vi "Bezier Trajectory.vi"(4 "Turn Rate":dbl=5.0 format="%#_13g", 5 "Max Robot Speed":dbl, 6 "Overrides":T3 {"Angle Override" step=5.0; "Velocity Override" step=5.0; "Angular Override" step=5.0}, 7 "Drive Type":T6, 8 "Conditions":T7, 9 "All Limits":cluster{"Limits":T4, "Angular Limits":T5} {"Limits"."StoopidFast (fps)" min=0.0; "Limits"."Jerk (fps^3)" min=0.0 step=1.0; "Limits"."Accel (fps^2)" min=0.0; "Limits"."Velocity (fps)" min=0.0; "Angular Limits"."Jerk (deg/s^3)" min=0.0 step=1.0; "Angular Limits"."Accel (deg/s^2)" min=0.0; "Angular Limits"."Velocity (deg/s)" min=0.0}, 10 "sample period (s)":sgl, 11 "WayPoints":T8) -> (0 "Time & Dist":cluster{"Time (s)":dbl, "Distance (ft)":dbl}, 1 "Valid":bool, 2 "Updated Waypoints":cluster{"x":dbl, "y":dbl, "th":dbl}[](array[cluster]), 3 "Trajectory Data":T2(array[cluster]))   [LabVIEW 2025]
uses:
  Types/Waypoints.ctl
  Types/Drive Type.ctl
  Types/Limits.ctl
  Types/Angluar Limits.ctl
  Types/Overrides.ctl
  Types/Segment Type.ctl
panel:
  out "XY Graph":cluster{"X":dbl, "Y":dbl}[](graph)
  in  "dynamic?":bool
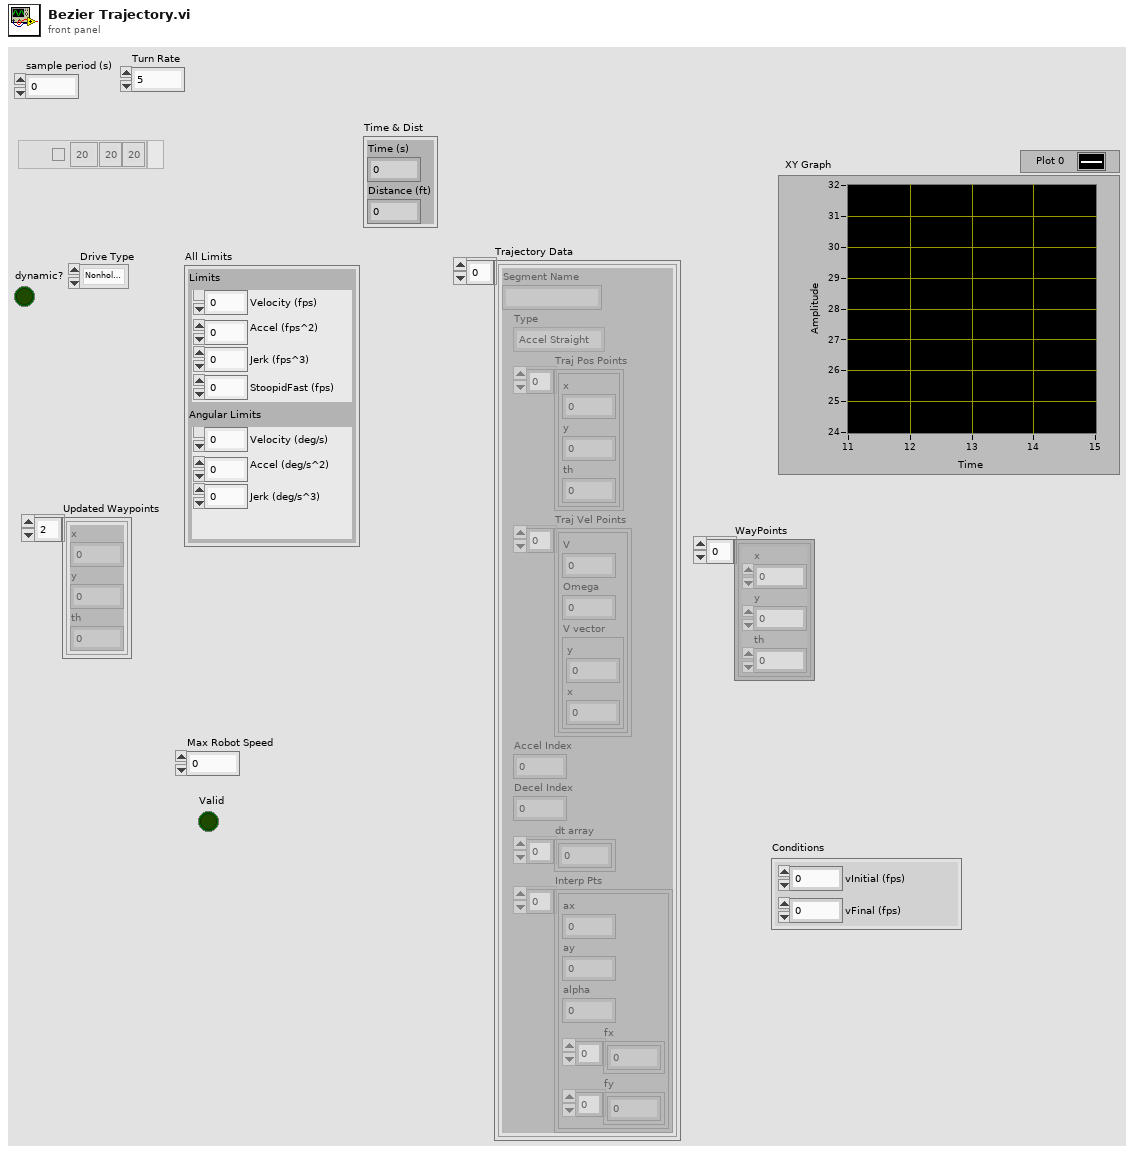
[diagram p1: front panel]
types:
  T1 = typedef "Segment Type.ctl" = enum16{"Accel Straight", "Const Straight", "Blend", "Circle", "Bezier", "Choreo"}
  T2 = cluster{"Segment Name":string, "Type":T1, "Traj Pos Points":cluster{"x":dbl, "y":dbl, "th":dbl}[], "Traj Vel Points":cluster{"V":dbl, "Omega":dbl, "V vector":cluster{"y":dbl, "x":dbl}}[], "Accel Index":i32, "Decel Index":i32, "dt array":dbl[], "Interp Pts":cluster{"ax":dbl, "ay":dbl, "alpha":dbl, "fx":dbl[], "fy":dbl[]}[]}[]
  T3 = typedef "Overrides.ctl" = cluster{"Count":string, "Angular Override":dbl, "Enabled?":bool, "Velocity Override":dbl, "Angle Override":dbl}[]
  T4 = typedef "Limits.ctl" = cluster{"Velocity (fps)":dbl, "Accel (fps^2)":dbl, "Jerk (fps^3)":dbl, "StoopidFast (fps)":dbl}
  T5 = typedef "Angluar Limits.ctl" = cluster{"Velocity (deg/s)":dbl, "Accel (deg/s^2)":dbl, "Jerk (deg/s^3)":dbl}
  T6 = typedef "Drive Type.ctl" = enum16{"Nonholonomic", "Holonomic"}
  T7 = cluster{"vInitial (fps)":dbl, "vFinal (fps)":dbl}
  T8 = typedef "Waypoints.ctl" = cluster{"x":sgl, "y":sgl, "th":sgl}[]
  T9 = cluster{"Segment Name":string, "Type":T1, "Traj Pos Points":cluster{"x":dbl, "y":dbl, "th":dbl}[], "Traj Vel Points":cluster{"V":dbl, "Omega":dbl, "V vector":cluster{"y":dbl, "x":dbl}}[], "Accel Index":i32, "Decel Index":i32, "dt array":dbl[], "Interp Pts":cluster{"ax":dbl, "ay":dbl, "alpha":dbl, "fx":dbl[], "fy":dbl[]}[]}
  T10 = cluster{"Velocity (fps)":dbl, "Accel (fps^2)":dbl, "Jerk (fps^3)":dbl}
  T11 = typedef "Bezier Curve.ctl" = cluster{"x":sgl, "y":sgl}[]
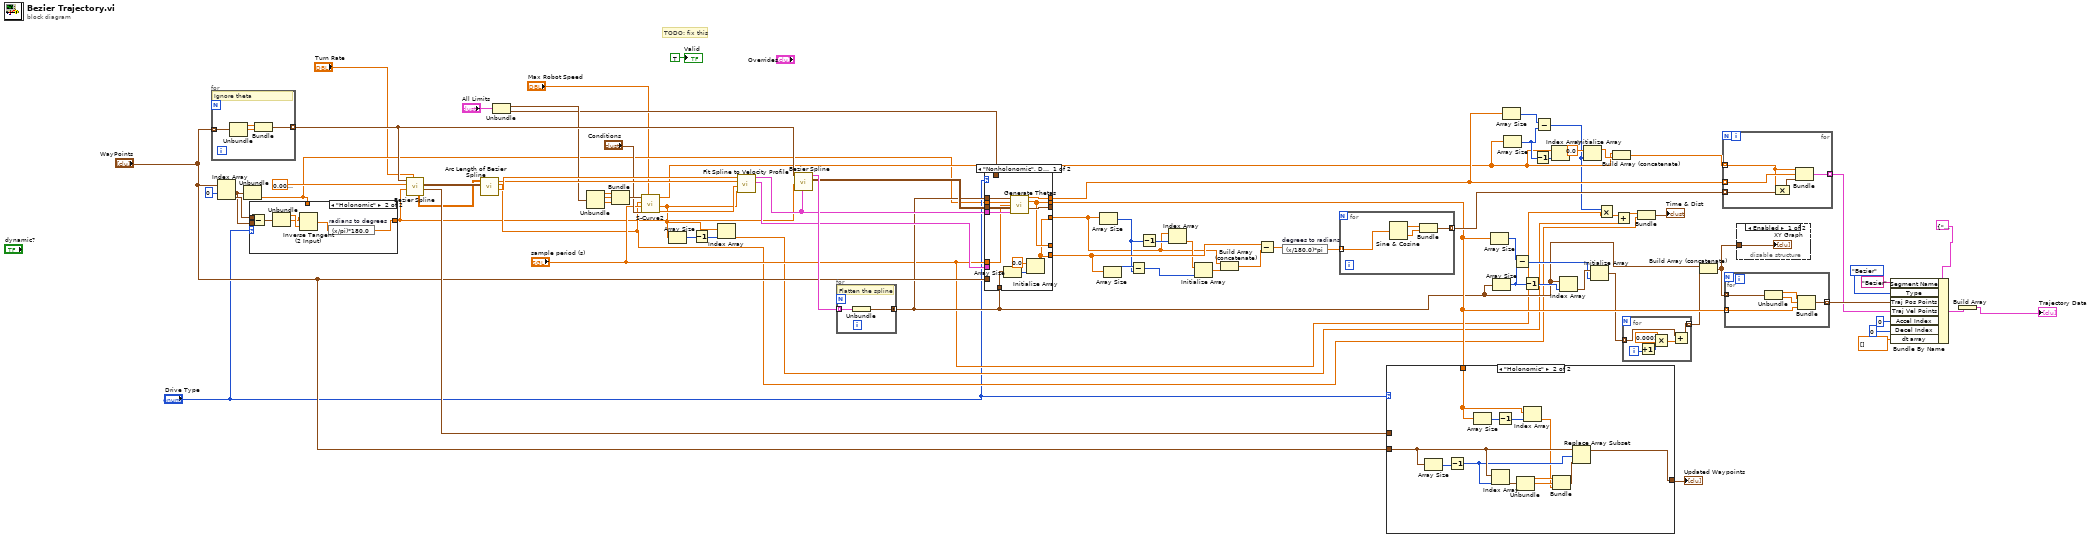
[diagram p0: block diagram]
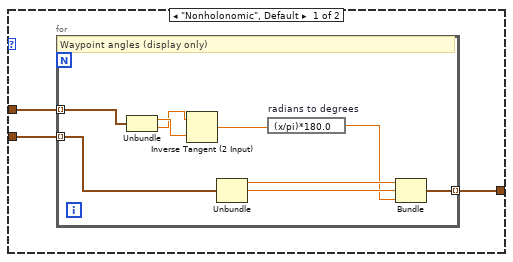
[diagram p4: hidden frame]
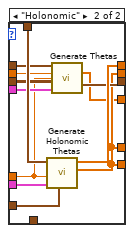
[diagram p5: hidden frame]
diagram:
  # "TODO: fix this"
  n1 = for {
    tunnel: "WayPoints" -> [w85] mode=indexing
    tunnel: [w82] -> w63 mode=indexing
    # "Ignore theta"
    n2 = Unbundle(w85) -> ("x"=w84:sgl, "y"=w83:sgl)  [unwired: 1 out]
    n3 = Bundle("x"=w84, "y"=w83) -> (w82:cluster{"x":sgl, "y":sgl})  [unwired: 1 in]
  }
  n4 = Index Array(array="WayPoints", index #1=0 ("index")) -> (element #1=w9:cluster{"x":sgl, "y":sgl, "th":sgl}, element #2=w10:cluster{"x":sgl, "y":sgl, "th":sgl})  [unwired: 1 in]
  n5 = Unbundle(w9) -> ("th"=w7:sgl)  [unwired: 2 out]
  n6 = case shown="\"Holonomic\"" "Drive Type" {
    tunnel: w10 -> [_ w93]
    tunnel: w9 -> [_ w92]
    tunnel: [w86 w87] -> w6
    tunnel: w7 -> [w86 _]
    frame "Nonholonomic", Default {
    }
    frame "Holonomic" {
      n7 = Subtract(x=w93, y=w92) -> (x-y=w91:cluster{"x":sgl, "y":sgl, "th":sgl})
      n8 = Unbundle(w91) -> ("x"=w90:sgl, "y"=w89:sgl)  [unwired: 1 out]
      n9 = Inverse Tangent (2 Input)(1:w90, 2:w89) -> (0:w88:sgl)
      n10 = expression code="(x/pi)*180.0" "radians to degrees"(w88) -> (w87:sgl)
    }
  }
  n11 = call "Bezier Spline.vi"("Turn Rate"="Turn Rate", "starting orientation (deg)"=w6, "percision"=sgl 0.01, "waypts"=w63) -> ("Tangents"=w76:cluster{sgl, sgl}[], "ctrl pts"=w66:cluster{sgl, sgl}[][], "position out"=w60:sgl[][])  [unwired: 3 in, 2 out]
  n12 = call "Arc Length of Bezier Spline.vi"("ctrl pts"=w66, "position"=w60) -> ("t"=w65:sgl[], "l total"=w13:dbl, "l"=w64:dbl[])  [unwired: 6 in, 1 out]
  n13 = Unbundle("All Limits") -> ("Limits"=w53:T4, "Angular Limits"=w52:T5)
  n14 = Unbundle(w53) -> ("Velocity (fps)"=w80:dbl, "Accel (fps^2)"=w79:dbl, "Jerk (fps^3)"=w78:dbl)  [unwired: 1 out]
  n15 = Bundle("Velocity (fps)"=w80, "Accel (fps^2)"=w79, "Jerk (fps^3)"=w78) -> (w77:T10)  [unwired: 1 in]
  n16 = call "S-Curve2.vi"("Max Robot Speed"="Max Robot Speed", "Conditions"="Conditions", "dt (s)"="sample period (s)", "goal"=w13, "Limits"=w77) -> ("X"=w62:dbl[], "T"=w56:dbl[], "V"=w23:dbl[])  [unwired: 4 in]
  n17 = Array Size(array=w56) -> (size(s)=w75:i32)
  n18 = Decrement(x=w75) -> (x-1=w74:i32)
  n19 = Index Array(array=w56, index=w74) -> (element=w14:dbl)
  n20 = call "Fit Spline to Velocity Profile.vi"("time"=w56, "vel positions"=w62, "s(t)"=w64, "t flat"=w65) -> ("time unflat"=w55:cluster{dbl[]}[], "y unflat"=w57:cluster{dbl[]}[])  [unwired: 6 in]
  n21 = call "Bezier Spline.vi"("positions"=w57, "starting orientation (deg)"=w6, "waypts"=w63) -> ("ctrl pts"=w58:cluster{sgl, sgl}[][], "bezier spline"=w59:cluster{"curve ":T11}[])  [unwired: 4 in, 3 out]
  n22 = for {
    tunnel: w59 -> [w95] mode=indexing
    tunnel: [w94] -> w39 mode=concatenating
    # "Flatten the spline"
    n23 = Unbundle(w95) -> ("curve"=w94:T11)
  }
  n24 = case shown="\"Nonholonomic\", Default" "Drive Type" {
    tunnel: [w107 w119] -> w29
    tunnel: [w101 w110] -> w45
    tunnel: w7 -> [w106 w114]
    tunnel: w39 -> [w105 w115]
    tunnel: w58 -> [w104 w113]
    tunnel: w57 -> [w103 w112]
    tunnel: w55 -> [_ w118]
    tunnel: "sample period (s)" -> [w96 w108]
    tunnel: w52 -> [_ w117]
    tunnel: "WayPoints" -> [_ w116]
    tunnel: [w102 w111] -> _
    tunnel: [w101 w110] -> _
    tunnel: [w97 w110] -> w38
    tunnel: [w97 w109] -> w32
    tunnel: w39 -> [w100 _]
    frame "Nonholonomic", Default {
      n25 = Array Size(array=w100) -> (size(s)=w99:i32)
      n26 = call "Generate Thetas.vi"("spline flat"=w105, "starting angle"=w106, "dt"=w96, "ctrl pts"=w104, "y unflat"=w103) -> ("omega"=w107:sgl[], "theta"=w101:sgl[], "Tangent Vector"=w102:cluster{"x out":dbl, "y out":dbl}[])  [unwired: 8 in]
      n27 = Initialize Array(0.0 ("element"), w99) -> (w97:dbl[])
    }
    frame "Holonomic" {
      n28 = call "Generate Holonomic Thetas.vi"("WayPoints"=w116, "time unflat"=w118, "dt"=w108, "Angular Limits"=w117) -> ("X"=w110:dbl[], "V"=w119:dbl[])  [unwired: 6 in]
      n29 = call "Generate Thetas.vi"("spline flat"=w115, "starting angle"=w114, "dt"=w108, "ctrl pts"=w113, "y unflat"=w112) -> ("theta"=w109:sgl[], "Tangent Vector"=w111:cluster{"x out":dbl, "y out":dbl}[])  [unwired: 8 in, 1 out]
    }
  }
  n30 = Array Size(array=w32) -> (size(s)=w35:i32)
  n31 = Array Size(array=w38) -> (size(s)=w37:i32)
  n32 = Subtract(x=w37, y=w35) -> (x-y=w36:i32)
  n33 = Decrement(x=w35) -> (x-1=w34:i32)
  n34 = Index Array(array=w32, index=w34) -> (element=w33:dbl)
  n35 = Initialize Array(w33, w36) -> (w31:dbl[])
  n36 = Build Array (concatenate)(w32, w31) -> (w30:dbl[])
  n37 = Subtract(x=w38, y=w30) -> (x-y=w46:dbl[])
  n38 = expression code="(x/180.0)*pi" "degrees to radians"(w46) -> (w47:dbl[])
  n39 = for {
    tunnel: w47 -> [w121] mode=indexing
    tunnel: [w123] -> w48 mode=indexing
    n40 = Sine & Cosine(0:w121) -> (1:w122:dbl, 2:w120:dbl)
    n41 = Bundle(w122, w120) -> (w123:cluster{dbl, dbl})  [unwired: 1 in]
  }
  n42 = case shown="\"Holonomic\"" "Drive Type" {
    tunnel: w76 -> [w126 _]
    tunnel: "WayPoints" -> [w125 w143]
    tunnel: [w124 w136] -> w51
    tunnel: w45 -> [_ w145]
    frame "Nonholonomic", Default {
      n43 = for {
        tunnel: w125 -> [w135] mode=indexing
        tunnel: w126 -> [w127] mode=indexing
        tunnel: [w132] -> w124 mode=indexing
        # "Waypoint angles (display only)"
        n44 = Unbundle(w127) -> (w130:sgl, w129:sgl)
        n45 = Inverse Tangent (2 Input)(1:w130, 2:w129) -> (0:w128:sgl)
        n46 = Unbundle(w135) -> ("x"=w134:sgl, "y"=w133:sgl)  [unwired: 1 out]
        n47 = expression code="(x/pi)*180.0" "radians to degrees"(w128) -> (w131:sgl)
        n48 = Bundle("x"=w134, "y"=w133, w131) -> (w132:cluster{"x":sgl, "y":sgl, sgl})  [unwired: 1 in]
      }
    }
    frame "Holonomic" {
      n49 = Array Size(array=w143) -> (size(s)=w144:i32)
      n50 = Decrement(x=w144) -> (x-1=w142:i32)
      n51 = Array Size(array=w145) -> (size(s)=w147:i32)
      n52 = Index Array(array=w143, index=w142) -> (element=w141:cluster{"x":sgl, "y":sgl, "th":sgl})
      n53 = Decrement(x=w147) -> (x-1=w146:i32)
      n54 = Unbundle(w141) -> ("x"=w140:sgl, "y"=w139:sgl)  [unwired: 1 out]
      n55 = Index Array(array=w145, index=w146) -> (element=w138:dbl)
      n56 = Bundle("x"=w140, "y"=w139, w138) -> (w137:cluster{"x":sgl, "y":sgl, dbl})  [unwired: 1 in]
      n57 = Replace Array Subset(array=w143, new element=w137, index=w142) -> (w136:T8)
    }
  }
  "Updated Waypoints" <- w51
  n58 = Array Size(array=w45) -> (size(s)=w44:i32)
  n59 = Array Size(array=w39) -> (size(s)=w43:i32)
  n60 = Array Size(array=w29) -> (size(s)=w28:i32)
  n61 = Array Size(array=w23) -> (size(s)=w27:i32)
  n62 = Subtract(x=w44, y=w43) -> (x-y=w40:i32)
  n63 = Decrement(x=w43) -> (x-1=w42:i32)
  n64 = Decrement(x=w27) -> (x-1=w26:i32)
  n65 = Subtract(x=w28, y=w27) -> (x-y=w19:i32)
  n66 = Index Array(array=w23, index=w26) -> ()  [unwired: 1 out]
  n67 = Index Array(array=w39, index=w42) -> (element=w41:cluster{"x":sgl, "y":sgl})
  n68 = Initialize Array(0.0 ("element"), w19) -> (w25:dbl[])
  n69 = Initialize Array(w41, w40) -> (w21:cluster{"x":sgl, "y":sgl}[])
  n70 = Multiply(x=w19, y="sample period (s)") -> (x*y=w18:sgl)
  n71 = Build Array (concatenate)(w23, w25) -> (w22:dbl[])
  n72 = Add(x=w18, y=w14) -> (x+y=w17:dbl)
  n73 = for {
    tunnel: w21 -> [w149] mode=indexing
    tunnel: [w148] -> w20 mode=indexing
    i -> [w152]
    n74 = Increment(x=w152) -> (x+1=w151:i32)
    n75 = Multiply(x=0.0001, y=w151) -> (x*y=w150:dbl)
    n76 = Add(x=w149, y=w150) -> (x+y=w148:cluster{"x":dbl, "y":dbl})
  }
  n77 = Bundle(w17, "l total"=w13) -> (→"Time & Dist":cluster{dbl, "l total":dbl})  [unwired: 1 in]
  n78 = Build Array (concatenate)(w39, w20) -> (w12:cluster{"x":dbl, "y":dbl}[])
  n79 = for {
    tunnel: w29 -> [w158] mode=indexing
    tunnel: w22 -> [w154] mode=indexing
    tunnel: [w157] -> w69 mode=indexing
    tunnel: w48 -> [w155] mode=indexing
    n80 = Compound Arithmetic op=MULTIPLY(w154, w155) -> (w156:cluster{dbl, dbl})
    n81 = Bundle("element"=w154, w158, w156) -> (w157:cluster{"element":dbl, dbl, cluster{dbl, dbl}})  [unwired: 1 in]
  }
  n82 = for {
    tunnel: w12 -> [w163] mode=indexing
    tunnel: [w160] -> w70 mode=indexing
    tunnel: w45 -> [w159] mode=indexing
    n83 = Unbundle(w163) -> ("x"=w162:dbl, "y"=w161:dbl)
    n84 = Bundle("x"=w162, "y"=w161, w159) -> (w160:cluster{"x":dbl, "y":dbl, dbl})  [unwired: 1 in]
  }
  n85 = disable-structure shown="Enabled" {
    disable-tunnel: w12 -> [w164 _]
    frame Enabled {
      "XY Graph" <- w164
    }
    frame Disabled {
    }
  }
  n86 = Bundle By Name(cluster=T9 {"Segment Name"="", "Type"=enum."Accel Straight", "Traj Pos Points"=[], "Traj Vel Points"=[], "Accel Index"=0, "Decel Index"=0, "dt array"=[], "Interp Pts"=[]}, "Segment Name"="Bezier", "Type"=Segment_Type."Bezier", "Traj Pos Points"=w70, "Traj Vel Points"=w69, "Accel Index"=0, "Decel Index"=0, "dt array"=dbl[] []) -> (w11:T9)
  n87 = Build Array(w11) -> (→"Trajectory Data":T2)
  "Valid" <- TRUE ("Valid")
